vi "Exponential Fit (obs).vi"(0 "Y":dbl[](array[numeric]), 1 "X":dbl[](array[numeric]), 2 "Standard Deviation":dbl[](array[numeric])) -> (3 "error":i32, 4 "Best Exponential Fit":dbl[](array[numeric]), 5 "amplitude":dbl, 6 "damping":dbl, 7 "mse":dbl)   [LabVIEW 2020, in "NI_AALPro.lvlib"]
uses:
  NI_AALPro.lvlib
  <resource>/lvanlys.dll
panel:
  # "This VI is obsolete !!!\nYou should replace this VI in your diagram with the Exponential Fit VI.  \n\nNOTE: If you have wired to the Standard Deviation input of this obsolete VI, \n           please be aware that the new Exponential Fit VI accepts a Weight \n           input instead of Standard Deviation. The equation that you can use to \n           map Standard Deviation to Weight is:\n\n             \t\tWeight = 1 / (Standard Deviation)^2"
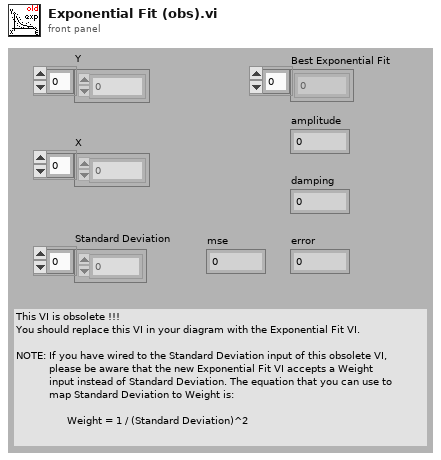
[diagram p1: front panel]
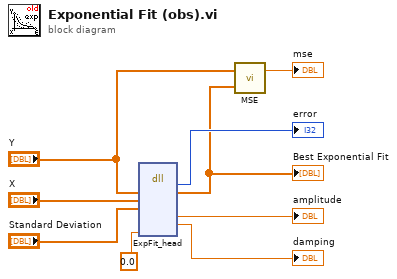
[diagram p0: block diagram]
diagram:
  n1 = dll-call lib="C:/Program Files (x86)/National Instruments/LabVIEW 2020/resource/lvanlys.*" fn="ExpFit_head"("y"="Y", "x"="X", "stdDev"="Standard Deviation", "mse"=0.0) -> (→"error":i32, "y"=w3:dbl[], "amp"=→"amplitude":dbl, "damping"=→"damping":dbl)  [unwired: 8 in, 2 out]
  "Best Exponential Fit" <- w3
  n2 = call "MSE.vi"("X Values"=w3, "Y Values"="Y") -> ("mse"=→"mse":dbl)  [unwired: 1 out]
